vi "c_Show.vi"() -> (1 "Case Label":T1)   [LabVIEW 2023, in "Worker-1.lvclass"]
uses:
  Worker-1.lvclass
  <vilib>/addons/_Workers/Library/Case Label.ctl
  <vilib>/addons/_Workers/Library/Workers.lvlib
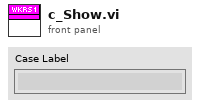
[diagram p1: front panel]
types:
  T1 = typedef "Workers.lvlib/Case Label.ctl" = string
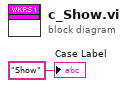
[diagram p0: block diagram]
diagram:
  "Case Label" <- T1 "Show" ("Case Label")
